vi "Dust Type Updater.vi"() -> ()   [LabVIEW 2012]
uses:
  <vilib>/addons/database/Connection.llb/Conn Execute.vi
  <vilib>/addons/database/Recordset.llb/Rec Fetch Recordset Data (R).vi
  <vilib>/addons/database/Recordset.llb/Rec Destroy - Connection.vi
  <userlib>/_OpenG.lib/array/array.llb/Remove Duplicates from 1D Array (String)__ogtk.vi
  <userlib>/_OpenG.lib/array/array.llb/Search 1D Array (String)__ogtk.vi
  <userlib>/_OpenG.lib/array/array.llb/Index 1D Array Elements (I32)__ogtk.vi
  <userlib>/_OpenG.lib/array/array.llb/Conditional Auto-Indexing Tunnel (I32)__ogtk.vi
  <userlib>/_OpenG.lib/comparison/comparison.llb/String Changed__ogtk.vi
  <userlib>/_OpenG.lib/comparison/comparison.llb/Variant Changed__ogtk.vi
  <userlib>/_OpenG.lib/array/array.llb/Index 1D Array Elements (DBL)__ogtk.vi
  <userlib>/_OpenG.lib/array/array.llb/Search 1D Array (I32)__ogtk.vi
  <userlib>/_OpenG.lib/array/array.llb/Filter 1D Array (I32)__ogtk.vi
  <vilib>/addons/database/_DB Variant To Data/Database Variant To Data.xnode
  <vilib>/addons/database/NI_Database_API.lvlib
panel:
  in  "New Dust":T1 {"New Batch" min=1 max=1 step=1; "New Type" min=1 max=1 step=1}
  out "Bottle Weights":dbl[](array[numeric])
  in  "Updateable Properties":T2
  in  "Create New Entry":bool
  in  "Cancel":bool
  in  "Update":bool
  in  "Update current entry":bool
  out "error IO":errorcluster
  in  "stop":bool
  out "Comments":string[](array[string])
  out "Dust Names":string[](array[string])
  out "Dust Weights":dbl[](array[numeric])
  out "Sizes":string[](array[string])
  out "Typical Weights":dbl[](array[numeric])
  out "Densities":dbl[](array[numeric])
  out "Batch Nos":i32[](array[numeric])
  out "Dust Type":i32[](array[numeric])
  out "Dust Type Ids":i32[](array[numeric])
  out "Dust Properties":T3
  in  "Dust":T4 {"Batch" min=1 max=1 step=1; "Type" min=1 max=1 step=1}
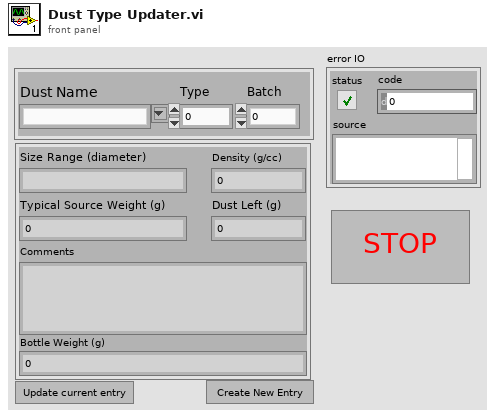
[diagram p1: front panel]
types:
  T1 = cluster{"New Dust Name":string, "New Type":u16, "New Batch":u16, "dust type id":u16, "Dust Left (g)":dbl, "Typical Source Weight (g)":dbl, "Density (g/cc)":dbl, "Size Range (diameter)":string, "Comments":string, "Bottle Weight (g)":dbl}
  T2 = cluster{"Size Range (diameter)":string, "Density (g/cc)":dbl, "Typical Source Weight (g)":dbl, "Tota lWeight (g)":dbl, "Comments":string, "Bottle Weight (g)":dbl}
  T3 = cluster{"Size Range (diameter)":string, "Density (g/cc)":dbl, "Typical Source Weight (g)":dbl, "Dust Left (g)":dbl, "Comments":string, "Bottle Weight (g)":dbl}
  T4 = cluster{"Dust Name":string, "Type":u16, "Batch":u16, "dust type id":u16}
  T5 = enum8{"Enabled", "Disabled", "Disabled and Grayed Out"}
  T6 = typedef "NI_Database_API.lvlib/Conn ObjectReference.ctl" = refnum<k1>
  T7 = typedef "NI_Database_API.lvlib/Rec ObjectReference.ctl" = refnum<k1>
  T8 = cluster{"data":string, "data":dbl, "data":dbl, "data":dbl, "data":string, "data":dbl}
  T9 = cluster{"data":string, "data":dbl, "data":dbl, dbl, "data":string, "data":dbl}
  T10 = cluster{"Size Range (diameter)":string, "Density (g/cc)":dbl, "Typical Source Weight (g)":dbl, dbl, "Comments":string, "Bottle Weight (g)":dbl}
  T11 = cluster{"Density (g/cc)":dbl, "Typical Source Weight (g)":dbl, "Size Range (diameter)":string, "Bottle Weight (g)":dbl, dbl, "Comments":string}
  T12 = cluster{"dust type id":u16, "New Dust Name":string, "New Type":u16, "New Batch":u16, "Density (g/cc)":dbl, "Typical Source Weight (g)":dbl, "Size Range (diameter)":string, "Bottle Weight (g)":dbl, "Dust Left (g)":dbl, "Comments":string}
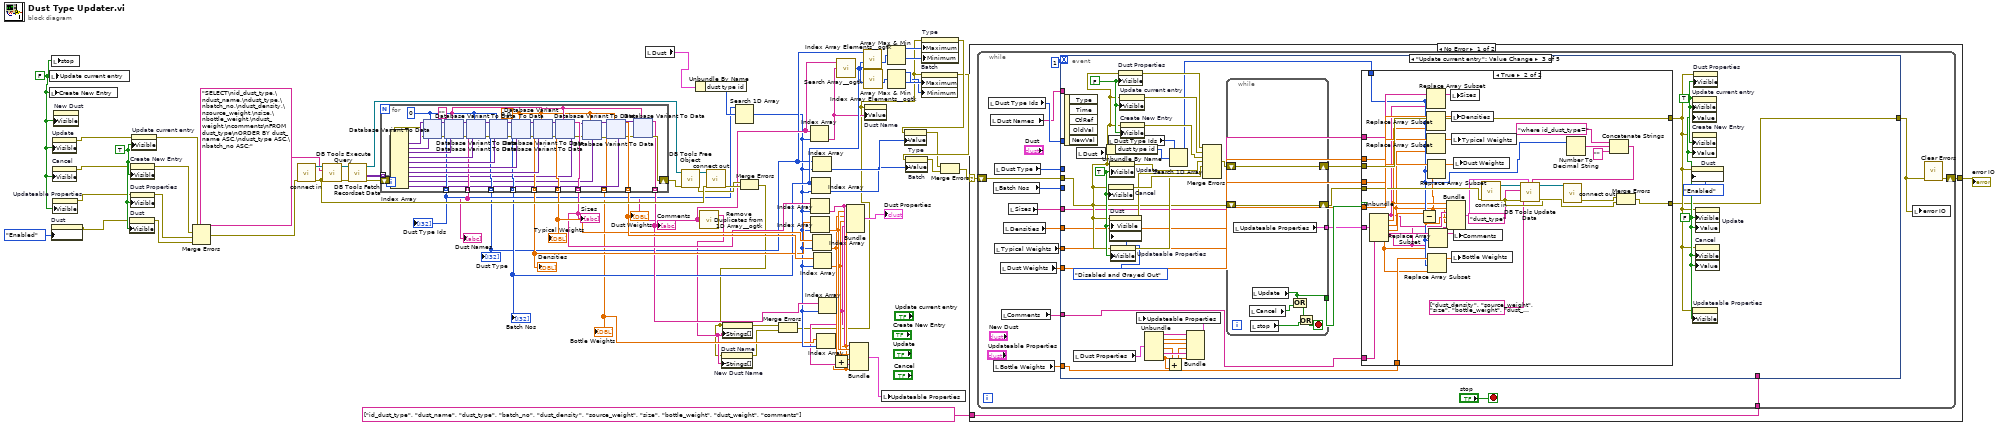
[diagram p0: block diagram]
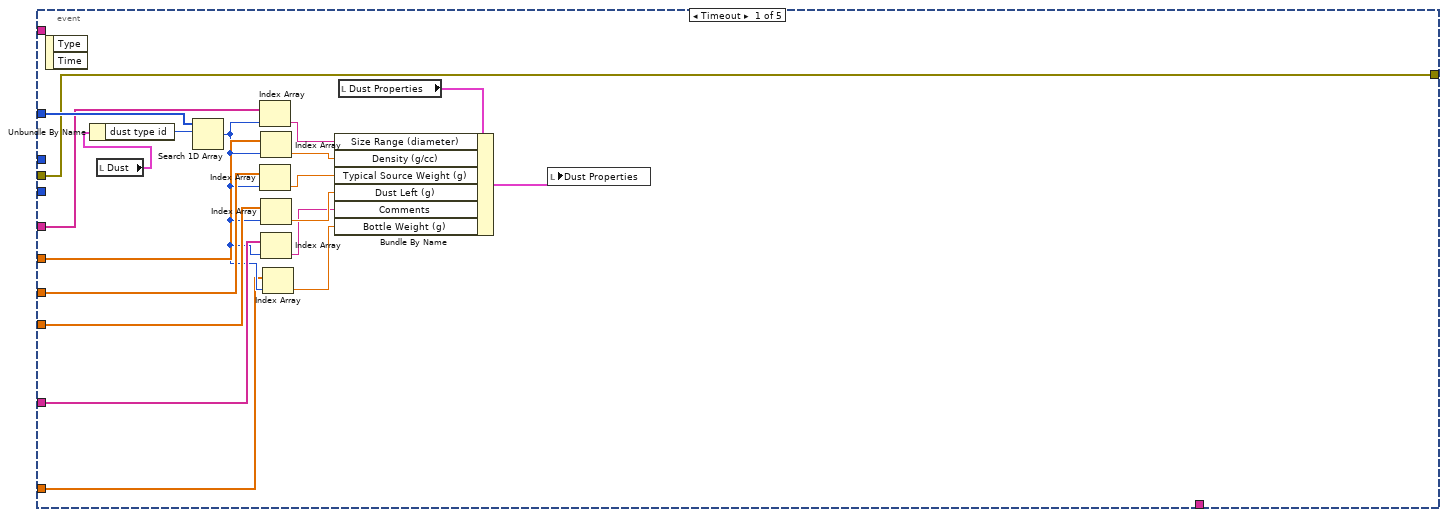
[diagram p2: hidden frame]
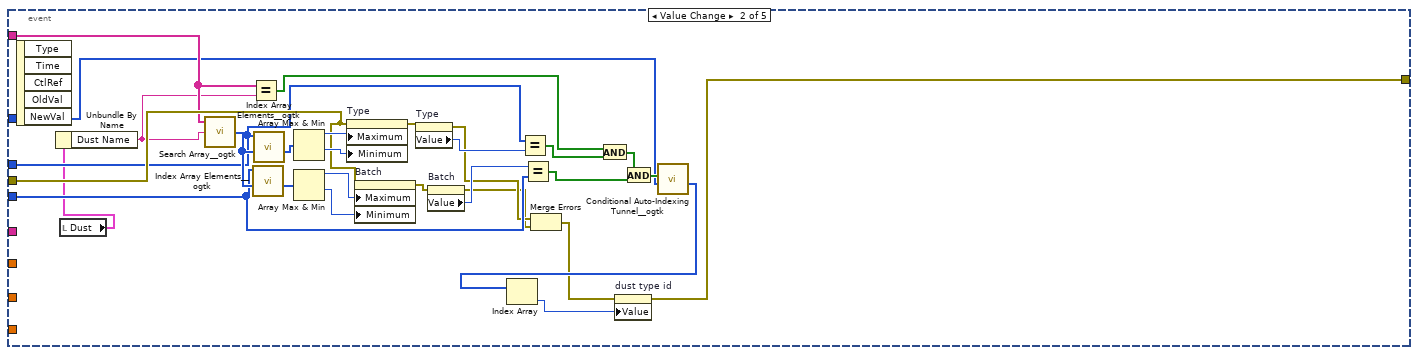
[diagram p3: hidden frame]
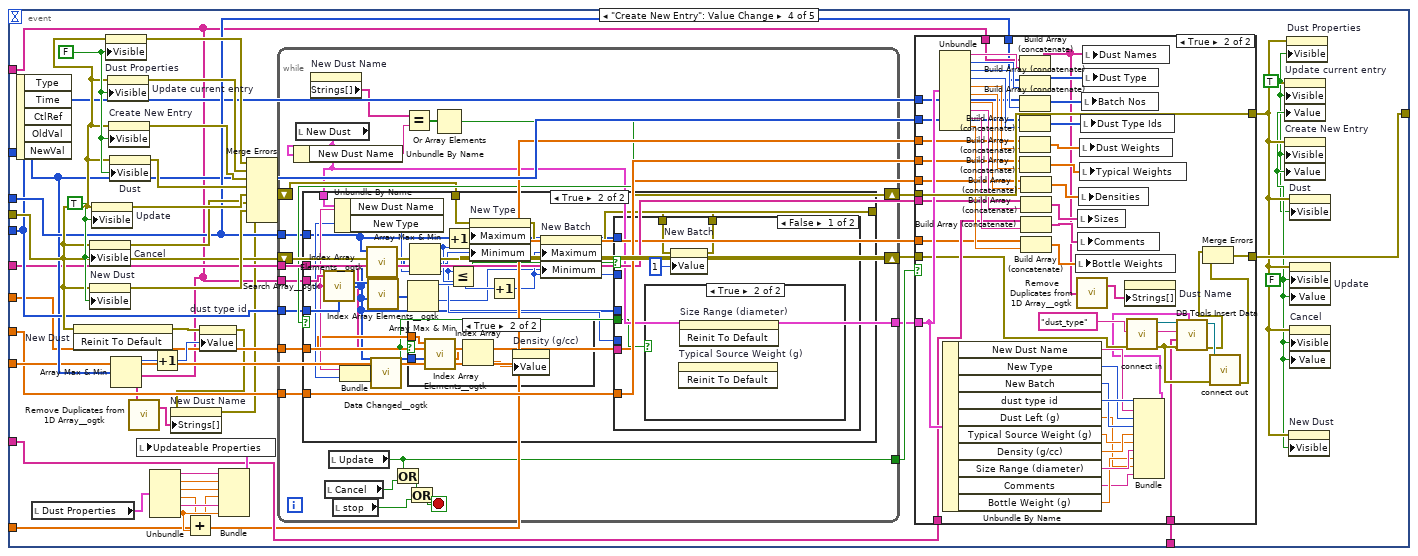
[diagram p5: hidden frame]
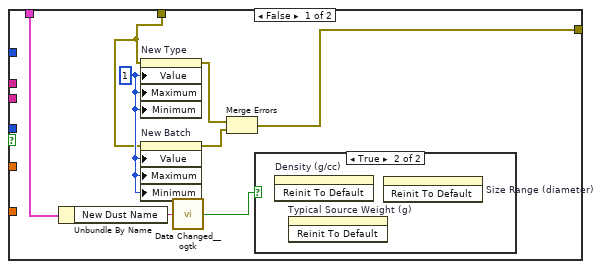
[diagram p7: hidden frame]
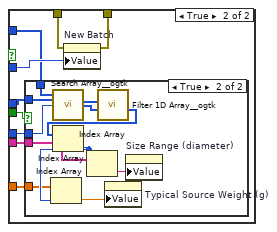
[diagram p11: hidden frame]
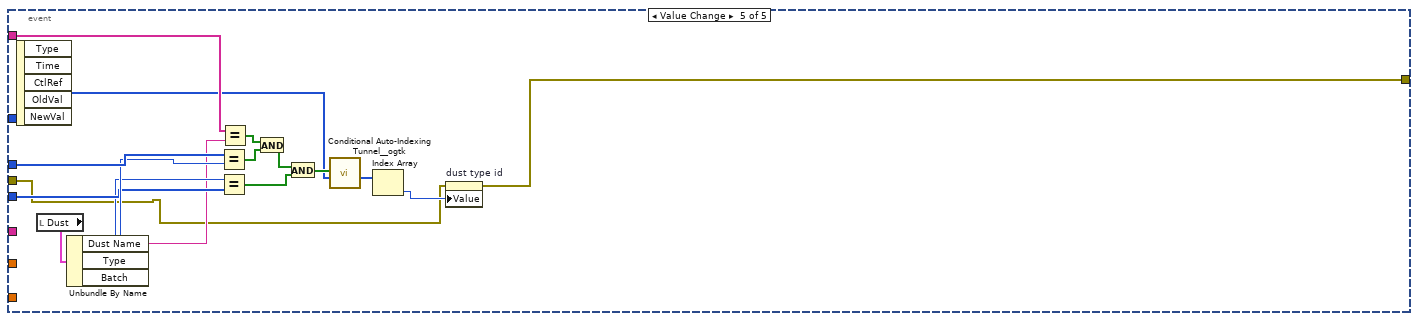
[diagram p13: hidden frame]
diagram:
  w29 = TRUE ("Visible")
  w7 = FALSE ("Update current entry")
  n1 = local write "Create New Entry"(w7) -> ()
  n2 = local write "Update current entry"(w7) -> ()
  n3 = property on="Dust" class="Clust (strict)"("DisabledEnum"=T5."Enabled" ("Disabled")) -> (error out=w20:errorcluster)  [unwired: 2 in, 1 out]
  n4 = local write "stop"(w7) -> ()
  n5 = property on="Update" class="Bool (strict)"("Visible"=w7) -> (error out=w26:errorcluster)  [unwired: 2 in, 1 out]
  n6 = property on="Cancel" class="Bool (strict)"("Visible"=w7) -> (error out=w27:errorcluster)  [unwired: 2 in, 1 out]
  n7 = property on="Updateable Properties" class="Clust (strict)"("Visible"=w7) -> (error out=w28:errorcluster)  [unwired: 2 in, 1 out]
  n8 = property on="New Dust" class="Clust (strict)"("Visible"=w7) -> ()  [unwired: 2 in, 2 out]
  n9 = property on="Dust" class="Clust (strict)"(error in=w20, "Visible"=w29) -> (error out=w21:errorcluster)  [unwired: 1 in, 1 out]
  n10 = property on="Create New Entry" class="Bool (strict)"(error in=w27, "Visible"=w29) -> (error out=w23:errorcluster)  [unwired: 1 in, 1 out]
  n11 = property on="Dust Properties" class="Clust (strict)"(error in=w28, "Visible"=w29) -> (error out=w22:errorcluster)  [unwired: 1 in, 1 out]
  n12 = property on="Update current entry" class="Bool (strict)"(error in=w26, "Visible"=w29) -> (error out=w24:errorcluster)  [unwired: 1 in, 1 out]
  n13 = Merge Errors(w24, w23, w22, w21) -> (w25:errorcluster)
  n14 = call "connect in.vi"("error in (no error)"=w25) -> ("error out"=w59:errorcluster, "Database Connection"=w66:T6)  [unwired: 6 in, 1 out]
  n15 = call-poly <vilib>:"DB Tools Execute Query.vi"("error in (no error)"=w59, "SQL query"="SELECT\nid_dust_type,\ndust_name,\ndust_type,\nbatch_no,\ndust_density,\nsource_weight,\nsize,\nbottle_weight,\ndust_weight,\ncomments\nFROM dust_type\nORDER BY dust_name ASC,\ndust_type ASC,\nbatch_no ASC;", "connection reference"=w66) -> ("error out"=w68:errorcluster, "recordset reference"=w67:T7)  [unwired: 5 in]
  n16 = call-poly <vilib>:"DB Tools Fetch Recordset Data.vi"("error in (no error)"=w68, "recordset reference"=w67) -> ("error out"=w63:errorcluster, "recordset data"=w64:variant[][], "recordset reference out"=w60:T7)  [unwired: 3 in]
  n17 = for {
    tunnel: w64 -> [w103] mode=indexing
    shift-right: [w77] -> w61
    shift-left: w63 -> [w95]
    tunnel: [w87] -> w50 mode=indexing
    tunnel: [w86] -> w46 mode=indexing
    tunnel: [w85] -> w43 mode=indexing
    tunnel: [w84] -> w44 mode=indexing
    tunnel: [w83] -> w54 mode=indexing
    tunnel: [w82] -> w55 mode=indexing
    tunnel: [w81] -> w53 mode=indexing
    tunnel: [w80] -> w56 mode=indexing
    tunnel: [w76] -> w52 mode=indexing
    tunnel: [w69] -> w17 mode=indexing
    w72 = 0.0
    w79 = ""
    w88 = 0
    n18 = Index Array(array=w103) -> (element #1=w102:variant, element #2=w101:variant, element #3=w100:variant, element #4=w99:variant, element #5=w98:variant, element #6=w97:variant, element #7=w96:variant, element #8=w73:variant, element #9=w74:variant, element #10=w75:variant)  [unwired: 10 in]
    n19 = xnode "Database Variant To Data"("database variant"=w102, "error in (no error)"=w95, "type"=w88) -> ("data"=w87:i32, "error out"=w94:errorcluster)
    n20 = xnode "Database Variant To Data"("database variant"=w101, "error in (no error)"=w94, "type"=w79) -> ("data"=w86:string, "error out"=w93:errorcluster)
    n21 = xnode "Database Variant To Data"("database variant"=w100, "error in (no error)"=w93, "type"=w88) -> ("data"=w85:i32, "error out"=w92:errorcluster)
    n22 = xnode "Database Variant To Data"("database variant"=w99, "error in (no error)"=w92, "type"=w88) -> ("data"=w84:i32, "error out"=w91:errorcluster)
    n23 = xnode "Database Variant To Data"("database variant"=w98, "error in (no error)"=w91, "type"=w72) -> ("data"=w83:dbl, "error out"=w90:errorcluster)
    n24 = xnode "Database Variant To Data"("database variant"=w97, "error in (no error)"=w90, "type"=w72) -> ("data"=w82:dbl, "error out"=w89:errorcluster)
    n25 = xnode "Database Variant To Data"("database variant"=w96, "error in (no error)"=w89, "type"=w79) -> ("data"=w81:string, "error out"=w71:errorcluster)
    n26 = xnode "Database Variant To Data"("database variant"=w73, "error in (no error)"=w71, "type"=w72) -> ("data"=w69:dbl, "error out"=w70:errorcluster)
    n27 = xnode "Database Variant To Data"("database variant"=w74, "error in (no error)"=w70, "type"=w72) -> ("data"=w80:dbl, "error out"=w78:errorcluster)
    n28 = xnode "Database Variant To Data"("database variant"=w75, "error in (no error)"=w78, "type"=w79) -> ("data"=w76:string, "error out"=w77:errorcluster)
  }
  "Dust Type Ids" <- w50
  "Dust Type" <- w43
  "Batch Nos" <- w44
  "Densities" <- w54
  "Typical Weights" <- w55
  "Sizes" <- w53
  "Dust Weights" <- w56
  "Dust Names" <- w46
  "Comments" <- w52
  "Bottle Weights" <- w17
  n29 = local read "Dust"() -> (w30:T4)
  n30 = call-poly <vilib>:"DB Tools Free Object.vi"("error in (no error)"=w61, "recordset reference"=w60) -> ("error out"=w57:errorcluster, "connection reference"=w62:T6)  [unwired: 8 in]
  n31 = Unbundle By Name(w30) -> ("dust type id"=w51:u16)
  n32 = call-poly <userlib>:"Remove Duplicates from 1D Array__ogtk.vi"("Input Array"=w46) -> ("Output Array"=w5:string[])  [unwired: 1 out]
  n33 = call "connect out.vi"("error in (no error)"=w59, "connection reference"=w62) -> ("error out"=w58:errorcluster)  [unwired: 9 in]
  n34 = Search 1D Array(1D array=w50, element=w51) -> (index of element=w18:i32)  [unwired: 1 in]
  n35 = Merge Errors(w57, w58) -> (w4:errorcluster)
  n36 = property on="New Dust Name" class="CmbBox"(error in=w4, "Strings[]"=w5) -> (error out=w2:errorcluster)  [unwired: 1 in, 1 out]
  n37 = property on="Dust Name" class="CmbBox"(error in=w4, "Strings[]"=w5) -> (error out=w34:errorcluster)  [unwired: 1 in, 1 out]
  n38 = Merge Errors(w34, w2) -> (w3:errorcluster)
  n39 = Index Array(array=w46, index=w18) -> (element=w6:string)
  n40 = Index Array(array=w53, index=w18) -> (element=w14:string)
  n41 = Index Array(array=w54, index=w18) -> (element=w13:dbl)
  n42 = Index Array(array=w44, index=w18) -> (element=w47:i32)
  n43 = Index Array(array=w43, index=w18) -> (element=w48:i32)
  n44 = Index Array(array=w55, index=w18) -> (element=w12:dbl)
  n45 = Index Array(array=w56, index=w18) -> (element=w11:dbl)
  n46 = Index Array(array=w17, index=w18) -> (element=w8:dbl)
  n47 = Index Array(array=w52, index=w18) -> (element=w10:string)
  n48 = Add(x=w11, y=w8) -> (x+y=w9:dbl)
  n49 = call-poly <userlib>:"Search Array__ogtk.vi"("Array"=w46, "Element Data"=w6) -> ("Indices of Elements"=w45:i32[])  [unwired: 7 in]
  n50 = Bundle("data"=w14, "data"=w13, "data"=w12, "data"=w11, "data"=w10, "data"=w8) -> (→"Dust Properties":T8)  [unwired: 1 in]
  n51 = Bundle("data"=w14, "data"=w13, "data"=w12, w9, "data"=w10, "data"=w8) -> (w15:T9)  [unwired: 1 in]
  n52 = call-poly <userlib>:"Index Array Elements__ogtk.vi"("indices"=w45, "array"=w43) -> ("elements"=w42:i32[])  [unwired: 9 in]
  n53 = call-poly <userlib>:"Index Array Elements__ogtk.vi"("indices"=w45, "array"=w44) -> ("elements"=w41:i32[])  [unwired: 9 in]
  n54 = property on="Dust Name" class="CmbBox"(error in=w3, "Value"=w6) -> ()  [unwired: 1 in, 2 out]
  n55 = local write "Updateable Properties"(w15) -> ()
  n56 = Array Max & Min(array=w42) -> (max value=w40:i32, min value=w39:i32)  [unwired: 2 out]
  n57 = Array Max & Min(array=w41) -> (max value=w38:i32, min value=w37:i32)  [unwired: 2 out]
  n58 = property on="Batch" class="DigNum (strict)"(error in=w3, "Maximum"=w38, "Minimum"=w37) -> (error out=w35:errorcluster)  [unwired: 1 in, 1 out]
  n59 = property on="Batch" class="DigNum (strict)"(error in=w35, "Value"=w47) -> (error out=w32:errorcluster)  [unwired: 1 in, 1 out]
  n60 = property on="Type" class="DigNum (strict)"(error in=w3, "Maximum"=w40, "Minimum"=w39) -> (error out=w36:errorcluster)  [unwired: 1 in, 1 out]
  n61 = property on="Type" class="DigNum (strict)"(error in=w36, "Value"=w48) -> (error out=w33:errorcluster)  [unwired: 1 in, 1 out]
  n62 = Merge Errors(w33, w32) -> (w31:errorcluster)
  n63 = case shown="No Error" w31 {
    selector: w31 -> [w426 w773]
    tunnel: [w425 w773] -> w49
    tunnel: string[] ["id_dust_type", "dust_name", "dust_type", "batch_no", "dust_density", "source_weight", "size", "bottle_weight", "dust_weight", "comments"] ("columns") -> [w424 _]
    frame No Error {
      n64 = while {
        shift-right: [w430] -> w425
        shift-left: w426 -> [w435]
        tunnel: w424 -> [w427]
        stop <- "stop" stop-if-true
        n65 = local read "Dust Type Ids"() -> (w441:i32[])
        n66 = local read "Dust Names"() -> (w434:string[])
        n67 = local read "Batch Nos"() -> (w432:i32[])
        n68 = local read "Bottle Weights"() -> (w428:dbl[])
        n69 = local read "Dust Type"() -> (w433:i32[])
        n70 = local read "Typical Weights"() -> (w438:dbl[])
        n71 = local read "Dust Weights"() -> (w437:dbl[])
        n72 = local read "Comments"() -> (w436:string[])
        n73 = local read "Densities"() -> (w439:dbl[])
        n74 = local read "Sizes"() -> (w440:string[])
        n75 = event shown="[2] \"Update current entry\": Value Change" {
          selector: _ -> [_ _ _ _ _]
          dyn-events: _ -> [_ _ _ _ _]
          timeout: 1 -> [_ _ _ _ _]
          tunnel: w441 -> [w460 w472 _ w588 w762]
          tunnel: w440 -> [w459 _ w494 w584 _]
          tunnel: w439 -> [w458 _ w495 w585 _]
          tunnel: w438 -> [w457 _ w496 w586 _]
          tunnel: w437 -> [w456 _ w497 w587 _]
          tunnel: w436 -> [w455 _ w498 w583 _]
          tunnel: w435 -> [w447 w485 w505 w594 w756]
          tunnel: [w447 w466 w503 w609 w759] -> w431
          tunnel: w434 -> [_ w482 _ w579 w772]
          tunnel: w433 -> [_ w480 _ w590 w771]
          tunnel: w432 -> [_ w479 _ w589 w769]
          tunnel: w428 -> [w444 _ w499 w582 _]
          tunnel: w427 -> [_ _ _ w577 _]
          event Timeout {
            n76 = event-data() -> ()  [unwired: 1 in, 2 out]
            n77 = local read "Dust"() -> (w446:T4)
            n78 = Unbundle By Name(w446) -> ("dust type id"=w461:u16)
            n79 = Search 1D Array(1D array=w460, element=w461) -> (index of element=w445:i32)  [unwired: 1 in]
            n80 = Index Array(array=w459, index=w445) -> (element=w454:string)
            n81 = Index Array(array=w457, index=w445) -> (element=w452:dbl)
            n82 = Index Array(array=w458, index=w445) -> (element=w453:dbl)
            n83 = Index Array(array=w456, index=w445) -> (element=w451:dbl)
            n84 = Index Array(array=w455, index=w445) -> (element=w450:string)
            n85 = Index Array(array=w444, index=w445) -> (element=w443:dbl)
            n86 = local read "Dust Properties"() -> (w448:T3)
            n87 = Bundle By Name(cluster=w448, "Size Range (diameter)"=w454, "Density (g/cc)"=w453, "Typical Source Weight (g)"=w452, "Dust Left (g)"=w451, "Comments"=w450, "Bottle Weight (g)"=w443) -> (w449:T3)
            n88 = local write "Dust Properties"(w449) -> ()
          }
          event "Dust.Dust Name": Value Change {
            n89 = event-data() -> ()  [unwired: 1 in, 5 out]
            n90 = local read "Dust"() -> (w465:T4)
            n91 = Unbundle By Name(w465) -> ("Dust Name"=w462:string)
            n92 = call-poly <userlib>:"Search Array__ogtk.vi"("Array"=w482, "Element Data"=w462) -> ("Indices of Elements"=w490:i32[])  [unwired: 7 in]
            n93 = Equal?(x=w482, y=w462) -> (x = y?=w476:bool[])
            n94 = call-poly <userlib>:"Index Array Elements__ogtk.vi"("indices"=w490, "array"=w479) -> ("elements"=w488:i32[])  [unwired: 9 in]
            n95 = call-poly <userlib>:"Index Array Elements__ogtk.vi"("indices"=w490, "array"=w480) -> ("elements"=w489:i32[])  [unwired: 9 in]
            n96 = Array Max & Min(array=w489) -> (max value=w487:i32, min value=w486:i32)  [unwired: 2 out]
            n97 = Array Max & Min(array=w488) -> (max value=w463:i32, min value=w464:i32)  [unwired: 2 out]
            n98 = property on="Type" class="DigNum (strict)"(error in=w485, "Maximum"=w487, "Minimum"=w486) -> (error out=w483:errorcluster)  [unwired: 1 in, 1 out]
            n99 = property on="Batch" class="DigNum (strict)"(error in=w485, "Maximum"=w463, "Minimum"=w464) -> (error out=w484:errorcluster)  [unwired: 1 in, 1 out]
            n100 = property on="Type" class="DigNum (strict)"(error in=w483) -> (error out=w469:errorcluster, "Value"=w481:u16)  [unwired: 1 in, 1 out]
            n101 = property on="Batch" class="DigNum (strict)"(error in=w484) -> (error out=w468:errorcluster, "Value"=w478:u16)  [unwired: 1 in, 1 out]
            n102 = Equal?(x=w480, y=w481) -> (x = y?=w477:bool[])
            n103 = Equal?(x=w478, y=w479) -> (x = y?=w474:bool[])
            n104 = Merge Errors(w469, w468) -> (w467:errorcluster)
            n105 = And(x=w476, y=w477) -> (x .and. y?=w475:bool[])
            n106 = And(x=w475, y=w474) -> (x .and. y?=w473:bool[])
            n107 = call-poly <userlib>:"Conditional Auto-Indexing Tunnel__ogtk.vi"("Array in"=w472, "Elements to keep"=w473) -> ("Filtered Array out"=w471:i32[])  [unwired: 5 in]
            n108 = Index Array(array=w471) -> (element=w470:i32)  [unwired: 1 in]
            n109 = property on="dust type id" class="Ring (strict)"(error in=w467, "Value"=w470) -> (error out=w466:errorcluster)  [unwired: 1 in, 1 out]
          }
          event "Update current entry": Value Change {
            w507 = FALSE ("Visible")
            w509 = TRUE ("Visible")
            w530 = TRUE ("Visible")
            w512 = FALSE ("Update current entry")
            n110 = event-data() -> ()  [unwired: 1 in, 5 out]
            n111 = local read "Dust Properties"() -> (w529:T3)
            n112 = local read "Dust"() -> (w524:T4)
            n113 = Unbundle By Name(w524) -> ("dust type id"=w523:u16)
            n114 = local read "Dust Type Ids"() -> (w522:i32[])
            n115 = property on="Cancel" class="Bool (strict)"(error in=w505, "Visible"=w530) -> (error out=w518:errorcluster)  [unwired: 1 in, 1 out]
            n116 = property on="Update" class="Bool (strict)"(error in=w505, "Visible"=w530) -> (error out=w519:errorcluster)  [unwired: 1 in, 1 out]
            n117 = property on="Dust" class="Clust (strict)"(error in=w505, "Visible"=w530, "DisabledEnum"=T5."Disabled and Grayed Out" ("Disabled")) -> (error out=w517:errorcluster)  [unwired: 1 in, 1 out]
            n118 = property on="Updateable Properties" class="Clust (strict)"(error in=w505, "Visible"=w530) -> (error out=w516:errorcluster)  [unwired: 1 in, 1 out]
            n119 = property on="Dust Properties" class="Clust (strict)"(error in=w505, "Visible"=w512) -> (error out=w511:errorcluster)  [unwired: 1 in, 1 out]
            n120 = property on="Update current entry" class="Bool (strict)"(error in=w505, "Visible"=w512) -> (error out=w521:errorcluster)  [unwired: 1 in, 1 out]
            n121 = property on="Create New Entry" class="Bool (strict)"(error in=w505, "Visible"=w512) -> (error out=w520:errorcluster)  [unwired: 1 in, 1 out]
            n122 = Unbundle(w529) -> ("Size Range (diameter)"=w528:string, "Density (g/cc)"=w527:dbl, "Typical Source Weight (g)"=w526:dbl, "Dust Left (g)"=w492:dbl, "Comments"=w525:string, "Bottle Weight (g)"=w493:dbl)
            n123 = Add(x=w492, y=w493) -> (x+y=w491:dbl)
            n124 = Search 1D Array(1D array=w522, element=w523) -> (index of element=w501:i32)  [unwired: 1 in]
            n125 = Bundle("Size Range (diameter)"=w528, "Density (g/cc)"=w527, "Typical Source Weight (g)"=w526, w491, "Comments"=w525, "Bottle Weight (g)"=w493) -> (w502:T10)  [unwired: 1 in]
            n126 = local write "Updateable Properties"(w502) -> ()
            n127 = Merge Errors(w511, w521, w520, w519, w518, w517, w516) -> (w515:errorcluster)
            n128 = while {
              shift-right: [w576] -> w513
              shift-left: w515 -> [w576]
              tunnel: [w575] -> w500
              tunnel: [w573] -> w514
              shift-right: [w572] -> w504
              shift-left: w505 -> [w572]
              stop <- w570 stop-if-true
              n129 = local read "Updateable Properties"() -> (w575:T2)
              n130 = local read "Cancel"() -> (w571:bool)
              n131 = local read "stop"() -> (w569:bool)
              n132 = local read "Update"() -> (w573:bool)
              n133 = Or(x=w573, y=w571) -> (x .or. y?=w574:bool)
              n134 = Or(x=w574, y=w569) -> (x .or. y?=w570:bool)
            }
            n135 = case shown="True" w514 {
              tunnel: w513 -> [w532 w568]
              tunnel: [w532 w568] -> w506
              tunnel: w504 -> [w531 w553]
              tunnel: [w531 w552] -> w503
              tunnel: w501 -> [_ w541]
              tunnel: w500 -> [_ w567]
              tunnel: w499 -> [_ w566]
              tunnel: w498 -> [_ w565]
              tunnel: w497 -> [_ w564]
              tunnel: w496 -> [_ w563]
              tunnel: w495 -> [_ w562]
              tunnel: w494 -> [_ w561]
              frame False {
              }
              frame True {
                n136 = Unbundle(w567) -> ("Size Range (diameter)"=w537:string, "Density (g/cc)"=w539:dbl, "Typical Source Weight (g)"=w538:dbl, "Tota lWeight (g)"=w554:dbl, "Comments"=w534:string, "Bottle Weight (g)"=w536:dbl)
                n137 = Subtract(x=w554, y=w536) -> (x-y=w535:dbl)
                n138 = Replace Array Subset(array=w561, new element=w537, index=w541) -> (w560:string[])
                n139 = Replace Array Subset(array=w562, new element=w539, index=w541) -> (w559:dbl[])
                n140 = Replace Array Subset(array=w563, new element=w538, index=w541) -> (w558:dbl[])
                n141 = Replace Array Subset(array=w564, new element=w535, index=w541) -> (w557:dbl[])
                n142 = Replace Array Subset(array=w566, new element=w536, index=w541) -> (w556:dbl[])
                n143 = Replace Array Subset(array=w565, new element=w534, index=w541) -> (w555:string[])
                n144 = Bundle("Density (g/cc)"=w539, "Typical Source Weight (g)"=w538, "Size Range (diameter)"=w537, "Bottle Weight (g)"=w536, w535, "Comments"=w534) -> (w533:T11)  [unwired: 1 in]
                n145 = local write "Sizes"(w560) -> ()
                n146 = local write "Densities"(w559) -> ()
                n147 = local write "Typical Weights"(w558) -> ()
                n148 = local write "Bottle Weights"(w556) -> ()
                n149 = local write "Comments"(w555) -> ()
                n150 = local write "Dust Weights"(w557) -> ()
                n151 = call "connect in.vi"("error in (no error)"=w553) -> ("error out"=w549:errorcluster, "Database Connection"=w547:T6)  [unwired: 6 in, 1 out]
                n152 = Number To Decimal String(number=w541) -> (decimal integer string=w543:string)  [unwired: 1 in]
                n153 = Concatenate Strings("where id_dust_type=" ("condition"), w543, "" ("string")) -> (w540:string)
                n154 = call <vilib>:"DB Tools Update Data.vi"("condition"=w540, "data"=w533, "error in (no error)"=w549, "columns"=string[] ["dust_density", "source_weight", "size", "bottle_weight", "dust_weight", "comments"], "table"="dust_type", "connection reference"=w547) -> ("error out"=w550:errorcluster, "connection reference out"=w546:T6)  [unwired: 4 in]
                n155 = call "connect out.vi"("error in (no error)"=w549, "connection reference"=w546) -> ("error out"=w551:errorcluster)  [unwired: 9 in]
                n156 = Merge Errors(w551, w550) -> (w552:errorcluster)
              }
            }
            n157 = property on="Dust" class="Clust (strict)"(error in=w506, "DisabledEnum"=T5."Enabled" ("Disabled")) -> ()  [unwired: 1 in, 2 out]
            n158 = property on="Update current entry" class="Bool (strict)"(error in=w506, "Visible"=w509, "Value"=w507) -> ()  [unwired: 1 in, 2 out]
            n159 = property on="Create New Entry" class="Bool (strict)"(error in=w506, "Visible"=w509, "Value"=w507) -> ()  [unwired: 1 in, 2 out]
            n160 = property on="Updateable Properties" class="Clust (strict)"(error in=w506, "Visible"=w507) -> ()  [unwired: 1 in, 2 out]
            n161 = property on="Dust Properties" class="Clust (strict)"(error in=w506, "Visible"=w509) -> ()  [unwired: 1 in, 2 out]
            n162 = property on="Update" class="Bool (strict)"(error in=w506, "Visible"=w507, "Value"=w507) -> ()  [unwired: 1 in, 2 out]
            n163 = property on="Cancel" class="Bool (strict)"(error in=w506, "Visible"=w507, "Value"=w507) -> ()  [unwired: 1 in, 2 out]
          }
          event "Create New Entry": Value Change {
            w597 = FALSE ("Visible")
            w596 = TRUE ("Visible")
            w603 = TRUE ("Visible")
            w604 = FALSE ("Update current entry")
            n164 = event-data() -> ()  [unwired: 1 in, 5 out]
            n165 = local read "Dust Properties"() -> (w621:T3)
            n166 = invoke on="New Dust" class="Clust (strict)" method="Reinit To Default"(error in=w594) -> (error out=w593:errorcluster)  [unwired: 2 in, 2 out]
            n167 = property on="Cancel" class="Bool (strict)"(error in=w594, "Visible"=w603) -> (error out=w600:errorcluster)  [unwired: 1 in, 1 out]
            n168 = property on="New Dust" class="Clust (strict)"(error in=w594, "Visible"=w603) -> (error out=w599:errorcluster)  [unwired: 1 in, 1 out]
            n169 = property on="Update" class="Bool (strict)"(error in=w594, "Visible"=w603) -> (error out=w601:errorcluster)  [unwired: 1 in, 1 out]
            n170 = property on="Dust Properties" class="Clust (strict)"(error in=w594, "Visible"=w604) -> (error out=w611:errorcluster)  [unwired: 1 in, 1 out]
            n171 = property on="Update current entry" class="Bool (strict)"(error in=w594, "Visible"=w604) -> (error out=w616:errorcluster)  [unwired: 1 in, 1 out]
            n172 = property on="Create New Entry" class="Bool (strict)"(error in=w594, "Visible"=w604) -> (error out=w615:errorcluster)  [unwired: 1 in, 1 out]
            n173 = property on="Dust" class="Clust (strict)"(error in=w594, "Visible"=w604) -> (error out=w602:errorcluster)  [unwired: 1 in, 1 out]
            n174 = Array Max & Min(array=w588) -> (max value=w592:i32)  [unwired: 3 out]
            n175 = call-poly <userlib>:"Remove Duplicates from 1D Array__ogtk.vi"("Input Array"=w579) -> ("Output Array"=w578:string[])  [unwired: 1 out]
            n176 = Unbundle(w621) -> ("Size Range (diameter)"=w620:string, "Density (g/cc)"=w619:dbl, "Typical Source Weight (g)"=w618:dbl, "Dust Left (g)"=w606:dbl, "Comments"=w617:string, "Bottle Weight (g)"=w607:dbl)
            n177 = Increment(x=w592) -> (x+1=w591:i32)
            n178 = Add(x=w606, y=w607) -> (x+y=w605:dbl)
            n179 = property on="dust type id" class="DigNum (strict)"(error in=w593, "Value"=w591) -> (error out=w581:errorcluster)  [unwired: 1 in, 1 out]
            n180 = property on="New Dust Name" class="CmbBox"(error in=w581, "Strings[]"=w578) -> (error out=w580:errorcluster)  [unwired: 1 in, 1 out]
            n181 = Bundle("Size Range (diameter)"=w620, "Density (g/cc)"=w619, "Typical Source Weight (g)"=w618, w605, "Comments"=w617, "Bottle Weight (g)"=w607) -> (w608:T10)  [unwired: 1 in]
            n182 = local write "Updateable Properties"(w608) -> ()
            n183 = Merge Errors(w611, w616, w615, w602, w601, w600, w599, w580) -> (w614:errorcluster)
            n184 = while {
              shift-right: [w681] -> w612
              shift-left: w614 -> [w682]
              tunnel: [w692] -> w613
              shift-right: [w693] -> w610
              shift-left: w594 -> [w693]
              tunnel: [w679] -> w595
              tunnel: w579 -> [w685]
              tunnel: w589 -> [w684]
              tunnel: w590 -> [w683]
              tunnel: w585 -> [w680]
              tunnel: w584 -> [w678]
              tunnel: w586 -> [w677]
              stop <- w691 stop-if-true
              n185 = local read "New Dust"() -> (w679:T1)
              n186 = Unbundle By Name(w679) -> ("New Dust Name"=w686:string)
              n187 = property on="New Dust Name" class="CmbBox"() -> ("Strings[]"=w689:string[])  [unwired: 2 in, 2 out]
              n188 = local read "Cancel"() -> (w695:bool)
              n189 = local read "Update"() -> (w692:bool)
              n190 = local read "stop"() -> (w690:bool)
              n191 = Or(x=w692, y=w695) -> (x .or. y?=w694:bool)
              n192 = Equal?(x=w689, y=w686) -> (x = y?=w688:bool[])
              n193 = Or(x=w694, y=w690) -> (x .or. y?=w691:bool)
              n194 = Or Array Elements(Boolean array=w688) -> (logical OR=w687:bool)
              n195 = case shown="True" w687 {
                tunnel: w685 -> [_ w728]
                tunnel: w684 -> [_ w727]
                tunnel: w683 -> [_ w708]
                tunnel: w682 -> [w702 w721]
                tunnel: [w699 w722] -> w681
                tunnel: w680 -> [_ w712]
                tunnel: w679 -> [w698 w715]
                tunnel: w678 -> [_ w707]
                tunnel: w677 -> [_ w706]
                frame False {
                  w703 = u16 1 ("Value")
                  n196 = Unbundle By Name(w698) -> ("New Dust Name"=w697:string)
                  n197 = property on="New Type" class="DigNum (strict)"(error in=w702, "Value"=w703, "Maximum"=w703, "Minimum"=w703) -> (error out=w701:errorcluster)  [unwired: 1 in, 1 out]
                  n198 = property on="New Batch" class="DigNum (strict)"(error in=w702, "Value"=w703, "Maximum"=w703, "Minimum"=w703) -> (error out=w700:errorcluster)  [unwired: 1 in, 1 out]
                  n199 = call-poly <userlib>:"Data Changed__ogtk.vi"("String"=w697) -> ("Changed"=w696:bool)
                  n200 = Merge Errors(w701, w700) -> (w699:errorcluster)
                  n201 = case shown="True" w696 {
                    frame False {
                    }
                    frame True {
                      n202 = invoke on="Density (g/cc)" class="DigNum (strict)" method="Reinit To Default"() -> ()  [unwired: 3 in, 3 out]
                      n203 = invoke on="Typical Source Weight (g)" class="DigNum (strict)" method="Reinit To Default"() -> ()  [unwired: 3 in, 3 out]
                      n204 = invoke on="Size Range (diameter)" class="Str" method="Reinit To Default"() -> ()  [unwired: 3 in, 3 out]
                    }
                  }
                }
                frame True {
                  n205 = Unbundle By Name(w715) -> ("New Dust Name"=w713:string, "New Type"=w710:u16)
                  n206 = call-poly <userlib>:"Search Array__ogtk.vi"("Array"=w728, "Element Data"=w713) -> ("Indices of Elements"=w709:i32[])  [unwired: 7 in]
                  n207 = Bundle("New Dust Name"=w713, "New Type"=w710) -> (w714:cluster{"New Dust Name":string, "New Type":u16})  [unwired: 1 in]
                  n208 = call-poly <userlib>:"Index Array Elements__ogtk.vi"("indices"=w709, "array"=w708) -> ("elements"=w726:i32[])  [unwired: 9 in]
                  n209 = call-poly <userlib>:"Index Array Elements__ogtk.vi"("indices"=w709, "array"=w727) -> ("elements"=w725:i32[])  [unwired: 9 in]
                  n210 = call-poly <userlib>:"Data Changed__ogtk.vi"("Variant"=w714) -> ("Changed"=w711:bool)
                  n211 = Array Max & Min(array=w725) -> (max value=w723:i32, min value=w704:i32)  [unwired: 2 out]
                  n212 = case shown="True" w711 {
                    tunnel: w712 -> [_ w731]
                    tunnel: w709 -> [_ w730]
                    frame False {
                    }
                    frame True {
                      n213 = call-poly <userlib>:"Index Array Elements__ogtk.vi"("indices"=w730, "array"=w731) -> ("elements"=w732:dbl[])  [unwired: 9 in]
                      n214 = Index Array(array=w732) -> (element=w729:dbl)  [unwired: 1 in]
                      n215 = property on="Density (g/cc)" class="DigNum (strict)"("Value"=w729) -> ()  [unwired: 2 in, 2 out]
                    }
                  }
                  n216 = Array Max & Min(array=w726) -> (max value=w720:i32, min value=w705:i32)  [unwired: 2 out]
                  n217 = Increment(x=w720) -> (x+1=w716:i32)
                  n218 = Less Or Equal?(x=w710, y=w720) -> (x <= y?=w724:bool)
                  n219 = property on="New Type" class="DigNum (strict)"(error in=w721, "Maximum"=w716, "Minimum"=w705) -> (error out=w719:errorcluster)  [unwired: 1 in, 1 out]
                  n220 = Increment(x=w723) -> (x+1=w717:i32)
                  n221 = property on="New Batch" class="DigNum (strict)"(error in=w719, "Maximum"=w717, "Minimum"=w704) -> (error out=w718:errorcluster)  [unwired: 1 in, 1 out]
                  n222 = case shown="False" w724 {
                    tunnel: w717 -> [_ w745]
                    tunnel: w718 -> [w735 w744]
                    tunnel: [w734 w743] -> w722
                    tunnel: w711 -> [w733 w742]
                    tunnel: w710 -> [_ w741]
                    tunnel: w709 -> [_ w740]
                    tunnel: w708 -> [_ w739]
                    tunnel: w707 -> [_ w738]
                    tunnel: w706 -> [_ w737]
                    frame False {
                      n223 = case shown="True" w733 {
                        frame False {
                        }
                        frame True {
                          n224 = invoke on="Typical Source Weight (g)" class="DigNum (strict)" method="Reinit To Default"() -> ()  [unwired: 3 in, 3 out]
                          n225 = invoke on="Size Range (diameter)" class="Str" method="Reinit To Default"() -> ()  [unwired: 3 in, 3 out]
                        }
                      }
                      n226 = property on="New Batch" class="DigNum (strict)"(error in=w735, "Value"=u16 1) -> (error out=w734:errorcluster)  [unwired: 1 in, 1 out]
                    }
                    frame True {
                      n227 = case shown="True" w742 {
                        tunnel: w741 -> [_ w753]
                        tunnel: w740 -> [_ w755]
                        tunnel: w739 -> [_ w754]
                        tunnel: w738 -> [_ w750]
                        tunnel: w737 -> [_ w748]
                        frame False {
                        }
                        frame True {
                          n228 = call-poly <userlib>:"Search Array__ogtk.vi"("Array"=w754, "Element Data"=w753) -> ("Indices of Elements"=w752:i32[])  [unwired: 7 in]
                          n229 = call-poly <userlib>:"Filter 1D Array__ogtk.vi"("items to filter"=w752, "array"=w755) -> ("filtered item indices"=w751:i32[])  [unwired: 4 in, 1 out]
                          n230 = Index Array(array=w751) -> (element=w749:i32)  [unwired: 1 in]
                          n231 = Index Array(array=w748, index=w749) -> (element=w746:dbl)
                          n232 = Index Array(array=w750, index=w749) -> (element=w747:string)
                          n233 = property on="Typical Source Weight (g)" class="DigNum (strict)"("Value"=w746) -> ()  [unwired: 2 in, 2 out]
                          n234 = property on="Size Range (diameter)" class="Str"("Value"=w747) -> ()  [unwired: 2 in, 2 out]
                        }
                      }
                      n235 = property on="New Batch" class="DigNum (strict)"(error in=w744, "Value"=w745) -> (error out=w743:errorcluster)  [unwired: 1 in, 1 out]
                    }
                  }
                }
              }
            }
            n236 = case shown="True" w613 {
              tunnel: w612 -> [w623 w676]
              tunnel: [w623 w676] -> w598
              tunnel: w610 -> [w622 w642]
              tunnel: [w622 w626] -> w609
              tunnel: w595 -> [_ w675]
              tunnel: w579 -> [_ w664]
              tunnel: w590 -> [_ w663]
              tunnel: w589 -> [_ w662]
              tunnel: w588 -> [_ w661]
              tunnel: w587 -> [_ w660]
              tunnel: w586 -> [_ w659]
              tunnel: w585 -> [_ w658]
              tunnel: w584 -> [_ w657]
              tunnel: w583 -> [_ w656]
              tunnel: w582 -> [_ w655]
              tunnel: w577 -> [_ w640]
              frame False {
              }
              frame True {
                n237 = Unbundle(w675) -> ("New Dust Name"=w674:string, "New Type"=w673:u16, "New Batch"=w672:u16, "dust type id"=w671:u16, "Dust Left (g)"=w670:dbl, "Typical Source Weight (g)"=w669:dbl, "Density (g/cc)"=w668:dbl, "Size Range (diameter)"=w667:string, "Comments"=w666:string, "Bottle Weight (g)"=w665:dbl)
                n238 = Unbundle By Name(w675) -> ("New Dust Name"=w636:string, "New Type"=w635:u16, "New Batch"=w634:u16, "dust type id"=w637:u16, "Dust Left (g)"=w629:dbl, "Typical Source Weight (g)"=w632:dbl, "Density (g/cc)"=w633:dbl, "Size Range (diameter)"=w631:string, "Comments"=w628:string, "Bottle Weight (g)"=w630:dbl)
                n239 = Build Array (concatenate)(w664, w674) -> (w645:string[])
                n240 = Build Array (concatenate)(w663, w673) -> (w654:i32[])
                n241 = Build Array (concatenate)(w662, w672) -> (w653:i32[])
                n242 = Build Array (concatenate)(w661, w671) -> (w652:i32[])
                n243 = Build Array (concatenate)(w660, w670) -> (w651:dbl[])
                n244 = Build Array (concatenate)(w659, w669) -> (w650:dbl[])
                n245 = Build Array (concatenate)(w658, w668) -> (w649:dbl[])
                n246 = Build Array (concatenate)(w657, w667) -> (w648:string[])
                n247 = Build Array (concatenate)(w656, w666) -> (w647:string[])
                n248 = Build Array (concatenate)(w655, w665) -> (w646:dbl[])
                n249 = local write "Bottle Weights"(w646) -> ()
                n250 = call-poly <userlib>:"Remove Duplicates from 1D Array__ogtk.vi"("Input Array"=w645) -> ("Output Array"=w644:string[])  [unwired: 1 out]
                n251 = local write "Sizes"(w648) -> ()
                n252 = local write "Comments"(w647) -> ()
                n253 = local write "Densities"(w649) -> ()
                n254 = local write "Dust Weights"(w651) -> ()
                n255 = local write "Typical Weights"(w650) -> ()
                n256 = local write "Dust Type Ids"(w652) -> ()
                n257 = local write "Batch Nos"(w653) -> ()
                n258 = local write "Dust Names"(w645) -> ()
                n259 = local write "Dust Type"(w654) -> ()
                n260 = property on="Dust Name" class="CmbBox"("Strings[]"=w644) -> ()  [unwired: 2 in, 2 out]
                n261 = call "connect in.vi"("error in (no error)"=w642) -> ("error out"=w641:errorcluster, "Database Connection"=w643:T6)  [unwired: 6 in, 1 out]
                n262 = Bundle("dust type id"=w637, "New Dust Name"=w636, "New Type"=w635, "New Batch"=w634, "Density (g/cc)"=w633, "Typical Source Weight (g)"=w632, "Size Range (diameter)"=w631, "Bottle Weight (g)"=w630, "Dust Left (g)"=w629, "Comments"=w628) -> (w627:T12)  [unwired: 1 in]
                n263 = call <vilib>:"DB Tools Insert Data.vi"("data"=w627, "error in (no error)"=w641, "columns"=w640, "table"="dust_type", "connection reference"=w643) -> ("error out"=w625:errorcluster, "connection reference out"=w638:T6)  [unwired: 5 in]
                n264 = call "connect out.vi"("error in (no error)"=w641, "connection reference"=w638) -> ("error out"=w624:errorcluster)  [unwired: 9 in]
                n265 = Merge Errors(w625, w624) -> (w626:errorcluster)
              }
            }
            n266 = property on="Update current entry" class="Bool (strict)"(error in=w598, "Visible"=w596, "Value"=w597) -> ()  [unwired: 1 in, 2 out]
            n267 = property on="Create New Entry" class="Bool (strict)"(error in=w598, "Visible"=w596, "Value"=w597) -> ()  [unwired: 1 in, 2 out]
            n268 = property on="Dust Properties" class="Clust (strict)"(error in=w598, "Visible"=w596) -> ()  [unwired: 1 in, 2 out]
            n269 = property on="New Dust" class="Clust (strict)"(error in=w598, "Visible"=w597) -> ()  [unwired: 1 in, 2 out]
            n270 = property on="Dust" class="Clust (strict)"(error in=w598, "Visible"=w596) -> ()  [unwired: 1 in, 2 out]
            n271 = property on="Update" class="Bool (strict)"(error in=w598, "Visible"=w597, "Value"=w597) -> ()  [unwired: 1 in, 2 out]
            n272 = property on="Cancel" class="Bool (strict)"(error in=w598, "Visible"=w597, "Value"=w597) -> ()  [unwired: 1 in, 2 out]
          }
          event "Dust.Type", "Dust.Batch": Value Change {
            n273 = event-data() -> ()  [unwired: 1 in, 5 out]
            n274 = local read "Dust"() -> (w758:T4)
            n275 = Unbundle By Name(w758) -> ("Dust Name"=w757:string, "Type"=w770:u16, "Batch"=w768:u16)
            n276 = Equal?(x=w771, y=w770) -> (x = y?=w766:bool[])
            n277 = Equal?(x=w768, y=w769) -> (x = y?=w764:bool[])
            n278 = Equal?(x=w772, y=w757) -> (x = y?=w767:bool[])
            n279 = And(x=w767, y=w766) -> (x .and. y?=w765:bool[])
            n280 = And(x=w765, y=w764) -> (x .and. y?=w763:bool[])
            n281 = call-poly <userlib>:"Conditional Auto-Indexing Tunnel__ogtk.vi"("Array in"=w762, "Elements to keep"=w763) -> ("Filtered Array out"=w761:i32[])  [unwired: 5 in]
            n282 = Index Array(array=w761) -> (element=w760:i32)  [unwired: 1 in]
            n283 = property on="dust type id" class="Ring (strict)"(error in=w756, "Value"=w760) -> (error out=w759:errorcluster)  [unwired: 1 in, 1 out]
          }
        }
        n284 = local write "error IO"(w431) -> ()
        n285 = call <vilib>:"Clear Errors.vi"("error in (no error)"=w431) -> ("error out"=w430:errorcluster)  [unwired: 6 in]
      }
    }
    frame Error {
    }
  }
  "error IO" <- w49
